vi "Trainer.vi"() -> ()   [LabVIEW 2021]
uses:
  <vilib>/Instr/_visa.llb/VISA Configure Serial Port (Instr).vi
panel:
  in  "stop":bool=TRUE
  out "Serial Settings:Number of Bytes at Serial Port":u32
  out "read buffer":string
  in  "VISA resource name":refnum<visa-resource-name>
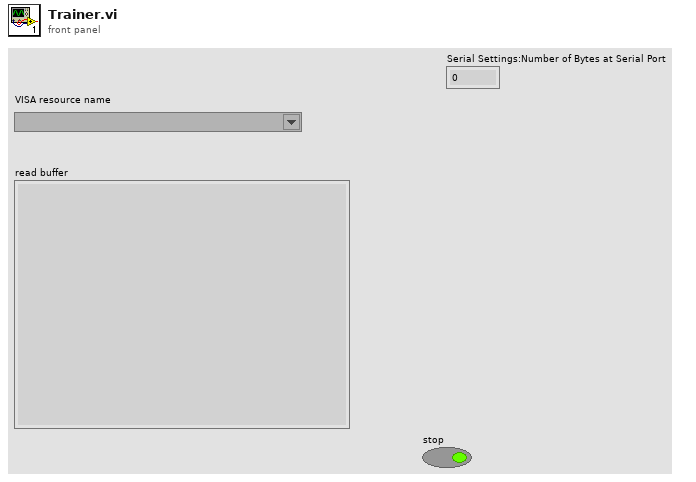
[diagram p1: front panel]
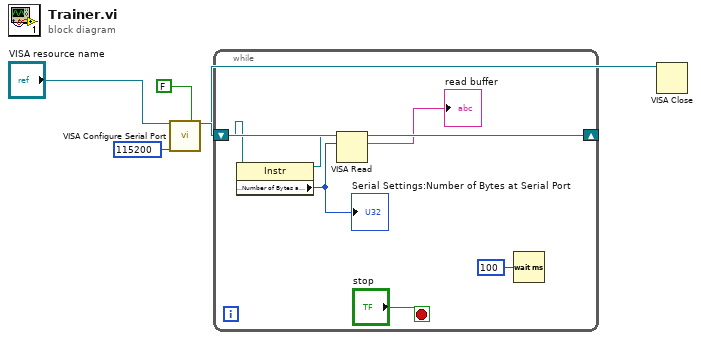
[diagram p0: block diagram]
diagram:
  n1 = call-poly "VISA Configure Serial Port"("VISA resource name"="VISA resource name", "Enable Termination\nChar (T)"=FALSE ("Enable Termination\nChar (T)"), "baud rate (9600)"=u32 115200) -> ("VISA resource name out"=w4:refnum<visa-resource-name>)  [unwired: 11 in, 1 out]
  n2 = while {
    shift-right: [w10] -> w3
    shift-left: w4 -> [w12]
    stop <- "stop" stop-if-true
    n3 = property class="Instr"(reference=w12) -> (reference out=w11:refnum<visa-resource-name>, "Serial Settings:Number of Bytes at Serial Port"=w9:u32)  [unwired: 1 in, 1 out]
    "Serial Settings:Number of Bytes at Serial Port" <- w9
    n4 = VISA Read(VISA resource name=w11, byte count=w9) -> (VISA resource name out=w10:refnum<visa-resource-name>, read buffer=→"read buffer":string)  [unwired: 1 in, 2 out]
    n5 = Wait (ms)(milliseconds to wait=u32 100) -> ()  [unwired: 1 out]
  }
  n6 = VISA Close(VISA resource name=w3) -> ()  [unwired: 1 in, 1 out]
